vi "Byte Order.vi"() -> (0 "Host byte order":T1, 1 "LabVIEW byte order":T1)   [LabVIEW 2027, in "Memory Manager.lvlib" / "Pointer.lvclass"]
doc: "Returns the bytes order for LabVIEW, which represents the byte order for strings returned from Type Cast, and the byte order for the host system."
uses:
  Pointer.lvclass
  Byte Order.ctl
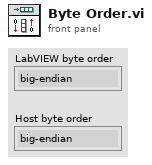
[diagram p1: front panel]
types:
  T1 = typedef "Memory Manager.lvlib/Pointer.lvclass/Byte Order.ctl" = enum8{"big-endian", "little-endian"}
  T2 = enum16{"big-endian, network order", "native, host order", "little-endian"}
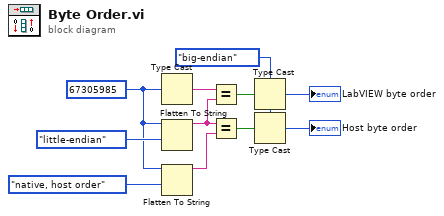
[diagram p0: block diagram]
diagram:
  w3 = Byte_Order."big-endian" ("byte order")
  w6 = u32 67305985
  n1 = Type Cast(x=w6) -> (*(type *) &x=w9:string)  [unwired: 1 in]
  n2 = Flatten To String(anything=w6, byte order (0:big-endian, network order)=T2."little-endian") -> (data string=w8:string)  [unwired: 2 in, 2 out]
  n3 = Flatten To String(anything=w6, byte order (0:big-endian, network order)=T2."native, host order") -> (data string=w7:string)  [unwired: 2 in, 2 out]
  n4 = Equal?(x=w9, y=w8) -> (x = y?=w4:bool)
  n5 = Equal?(x=w8, y=w7) -> (x = y?=w5:bool)
  n6 = Type Cast(type=w3, x=w4) -> (*(type *) &x=→"LabVIEW byte order":T1)
  n7 = Type Cast(type=w3, x=w5) -> (*(type *) &x=→"Host byte order":T1)
